vi "test_log.vi"() -> ()   [LabVIEW 2017]
uses:
  Logging/Logging.lvlib
panel:
  out "error out":errorcluster
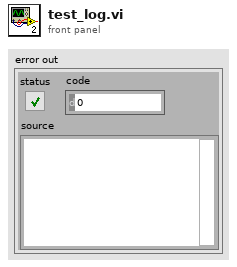
[diagram p1: front panel]
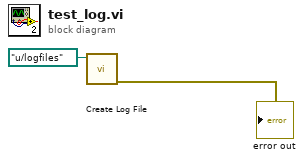
[diagram p0: block diagram]
diagram:
  n1 = call "Create Log File.vi"("Acceleration Exceeded Log Folder"=path "u:/logfiles") -> ("error out"=→"error out":errorcluster)  [unwired: 9 in, 1 out]
